vi "AlliGator Get Pile-up Correction Parameter.vi"(8 "error in (no error)":errorcluster, 9 "Pixel Well Capacity in":u32, 10 "Pile-up Correction in":bool, 11 "Data Information":string) -> (0 "error out":errorcluster, 1 "Pixel Well Capacity out":u32, 2 "Pile-up Correction out":bool, 3 "Pile-up Correction (already) applied?":bool)   [LabVIEW 2021, in "AlliGator HDF5.lvlib"]
doc: "Reads from the metadata whether or not pile-up correction was already applied, and if so, does not repeat it."
uses:
  AlliGator HDF5.lvlib
panel:
  # "see the AlliGator License on the block diagram (Ctrl+E or Window:Show Block Diagram)"
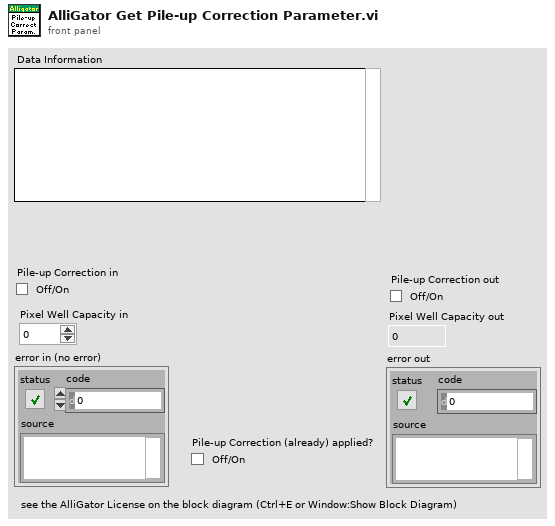
[diagram p1: front panel]
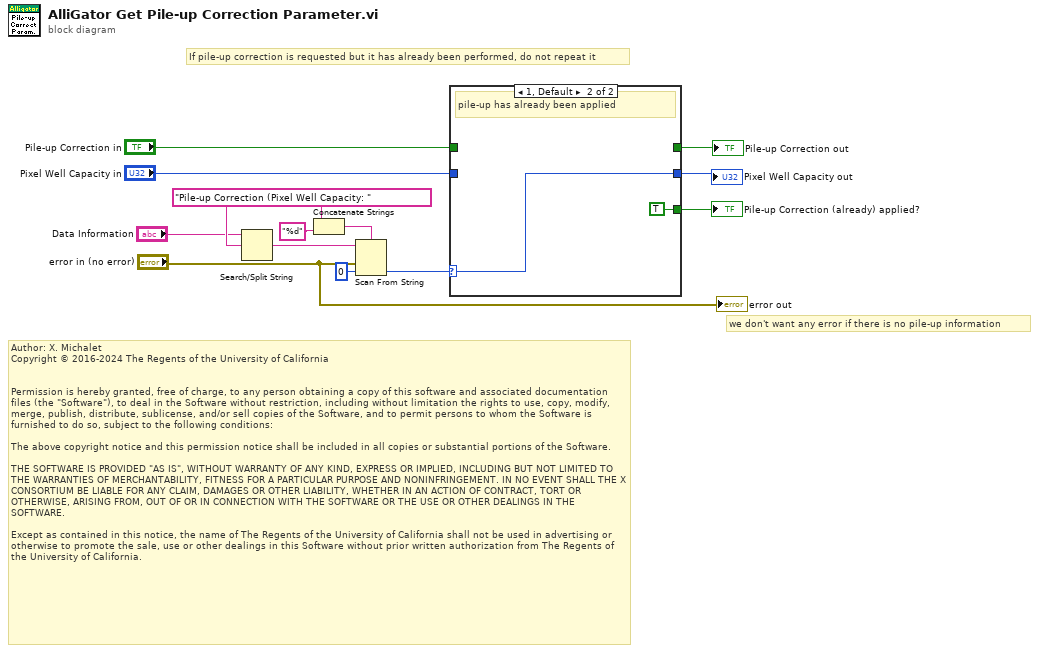
[diagram p0: block diagram]
diagram:
  w11 = "Pile-up Correction (Pixel Well Capacity: " ("format string")
  # "Author: X. Michalet\nCopyright © 2016-2024 The Regents of the University of California\n \n\nPermission is hereby granted, free of charge, to any person obtaining a copy of this software and associated documentation files (the \"Software\"), to deal in the Software without restriction, including without limitation the rights to use, copy, modify, merge, publish, distribute, sublicense, and/or sell copies of the Software, and to permit persons to whom the Software is furnished to do so, subject to the following conditions:\n\nThe above copyright notice and this permission notice shall be included in all copies or substantial portions of the Software.\n\nTHE SOFTWARE IS PROVIDED \"AS IS\", WITHOUT WARRANTY OF ANY KIND, EXPRESS OR IMPLIED, INCLUDING BUT NOT LIMITED TO THE WARRANTIES OF MERCHANTABILITY, FITNESS FOR A PARTICULAR PURPOSE AND NONINFRINGEMENT. IN NO EVENT SHALL THE X CONSORTIUM BE LIABLE FOR ANY CLAIM, DAMAGES OR OTHER LIABILITY, WHETHER IN AN ACTION OF CONTRACT, TORT OR OTHERWISE, ARISING FROM, OUT OF OR IN CONNECTION WITH THE SOFTWARE OR THE USE OR OTHER DEALINGS IN THE SOFTWARE.\n\nExcept as contained in this notice, the name of The Regents of the University of California shall not be used in advertising or otherwise to promote the sale, use or other dealings in this Software without prior written authorization from The Regents of the University of California."
  # "If pile-up correction is requested but it has already been performed, do not repeat it"
  # "we don't want any error if there is no pile-up information"
  n1 = Search/Split String(string="Data Information", search string/char (-)=w11) -> (match + rest of string=w9:string)  [unwired: 1 in, 2 out]
  n2 = Concatenate Strings(w11, "%d" ("string")) -> (w13:string)
  n3 = Scan From String(format string=w13, input string=w9, error in="error in (no error)", default 1=u32 0 ("default value 1")) -> (output 1=w6:u32)  [unwired: 1 in, 3 out]
  n4 = case shown="1, Default" w6 {
    selector: w6 -> [_ w17]
    tunnel: "Pile-up Correction in" -> [w14 _]
    tunnel: [w14 _] -> w4
    tunnel: "Pixel Well Capacity in" -> [w15 _]
    tunnel: [w15 w17] -> w2
    tunnel: [w14 TRUE ("Pile-up Correction in")] -> w1
    frame 0 {
      # "pile-up was not applied"
    }
    frame 1, Default {
      # "pile-up has already been applied"
    }
  }
  "Pixel Well Capacity out" <- w2
  "Pile-up Correction out" <- w4
  "Pile-up Correction (already) applied?" <- w1
  "error out" <- "error in (no error)"
